vi "Read Sensor.vi"(0 "VISA resource name":refnum<visa-resource-name>, 7 "Input (0: A)":u16(ring) items=["A", "B"], 11 "error in (no error)":errorcluster) -> (4 "VISA resource name out":refnum<visa-resource-name>, 6 "Celsius Reading":dbl min=-273.16 max=1372.0 step=1e-05 format="%^.5e", 8 "Kelvin Reading":dbl min=0.0 max=1645.0 step=1e-05 format="%^.5e", 10 "Sensor Units Reading":dbl min=-7.5 max=300000.0 step=1e-05 format="%^.5e", 15 "error out":errorcluster)   [LabVIEW 2014, in "Lake Shore Cryotronics 331.lvlib"]
doc: "This VI querys the instrument for an inputs sensor reading in Celsius, Kelvin, and Sensor Units."
uses:
  Lake Shore Cryotronics 331.lvlib
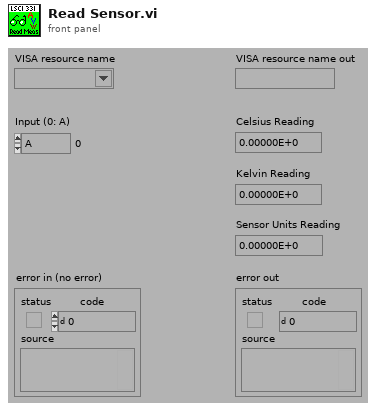
[diagram p1: front panel]
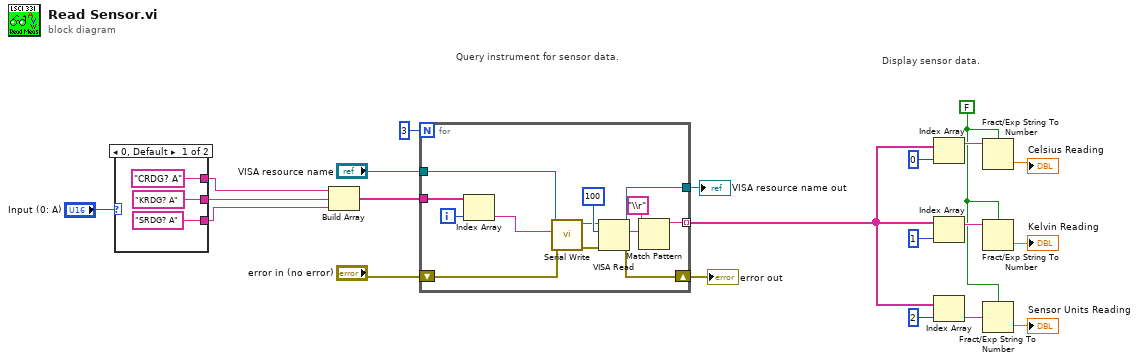
[diagram p0: block diagram]
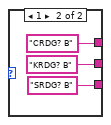
[diagram p2: hidden frame]
diagram:
  w5 = FALSE ("use system decimal point (T)")
  # "Query instrument for sensor data."
  # "Display sensor data."
  n1 = case shown="0, Default" "Input (0: A)" {
    tunnel: ["KRDG? A" "KRDG? B"] -> w3
    tunnel: ["CRDG? A" "CRDG? B"] -> w2
    tunnel: ["SRDG? A" "SRDG? B"] -> w1
    frame 0, Default {
    }
    frame 1 {
    }
  }
  n2 = Build Array(w2, w3, w1) -> (w12:string[])
  n3 = for {
    N: 3 -> [_]
    tunnel: w12 -> [w37]
    shift-right: [w34] -> w8
    shift-left: "error in (no error)" -> [w35]
    tunnel: [w33] -> w7
    tunnel: "VISA resource name" -> [w32]
    tunnel: [w30] -> w6 mode=indexing
    i -> [w36]
    n4 = Index Array(array=w37, index=w36) -> (element=w28:string)
    n5 = call "Serial Write.vi"("error in (no error)"=w35, "Write Buffer (\"\")"=w28, "VISA resource name"=w32) -> ("error out"=w40:errorcluster, "VISA resource name out"=w29:refnum<visa-resource-name>)  [unwired: 6 in, 1 out]
    n6 = VISA Read(VISA resource name=w29, byte count=100, error in (no error)=w40) -> (VISA resource name out=w33:refnum<visa-resource-name>, read buffer=w38:string, error out=w34:errorcluster)  [unwired: 1 out]
    n7 = Match Pattern(string=w38, regular expression="\\r") -> (before substring=w30:string)  [unwired: 1 in, 3 out]
  }
  "VISA resource name out" <- w7
  "error out" <- w8
  n8 = Index Array(array=w6, index=0) -> (element=w16:string)
  n9 = Index Array(array=w6, index=1) -> (element=w17:string)
  n10 = Index Array(array=w6, index=2) -> (element=w18:string)
  n11 = Fract/Exp String To Number(use system decimal point (T)=w5, string=w16) -> (number=→"Celsius Reading":dbl)  [unwired: 2 in, 1 out]
  n12 = Fract/Exp String To Number(use system decimal point (T)=w5, string=w17) -> (number=→"Kelvin Reading":dbl)  [unwired: 2 in, 1 out]
  n13 = Fract/Exp String To Number(use system decimal point (T)=w5, string=w18) -> (number=→"Sensor Units Reading":dbl)  [unwired: 2 in, 1 out]
